vi "DSF.Transceiver.GE Reflective Memory.Initialize Transfer Parameters.vi"(8 "error in (no error)":errorcluster, 10 "Transfer Configurations":refnum<class "DSF.Shared.Configuration.Transfer.lvclass">[](array[class]), 11 "DSF GE Reflective Memory Transceiver in":refnum<class "DSF.Transceiver.GE Reflective Memory.lvclass">) -> (0 "error out":errorcluster, 2 "Transfers Parameters":T1[](array[typedef]) {"size" format="%d bytes"; "offset" format="%08x"}, 3 "DSF GE Reflective Memory Transceiver out":refnum<class "DSF.Transceiver.GE Reflective Memory.lvclass">)   [LabVIEW 2017, in "DSF.Transceiver.GE Reflective Memory.lvlib" / "DSF.Transceiver.GE Reflective Memory.lvclass"]
uses:
  DSF.Transceiver.GE Reflective Memory.lvclass
  DSF Core/Built/Engine/DSF.Engine.lvlibp/Shared/Classes/Transfer/DSF.Shared.Configuration.Transfer.lvclass
  DSF.Transceiver.GE Reflective Memory.Transfer Parameters.ctl
  DSF Core/Built/Engine/DSF.Engine.lvlibp/Shared/Classes/Configuration/DSF.Shared.Configuration.lvclass
  C:/Git/DSF/DSF Core/Built/Engine/DSF.Engine.lvlibp/Shared/Classes/Configuration/DSF.Shared.Configuration.lvclass
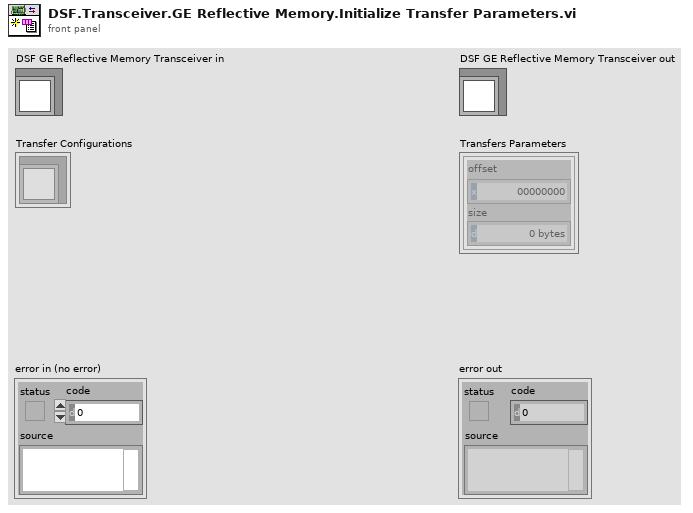
[diagram p1: front panel]
types:
  T1 = typedef "DSF.Transceiver.GE Reflective Memory.lvlib/DSF.Transceiver.GE Reflective Memory.lvclass/DSF.Transceiver.GE Reflective Memory.Transfer Parameters.ctl" = cluster{"offset":u32, "size":u32}
  T2 = typedef "DSF.Engine.lvlibp/DSF Configuration API.lvlib/DSF Settings Info.ctl" = cluster{"key":string, "value":string}[]
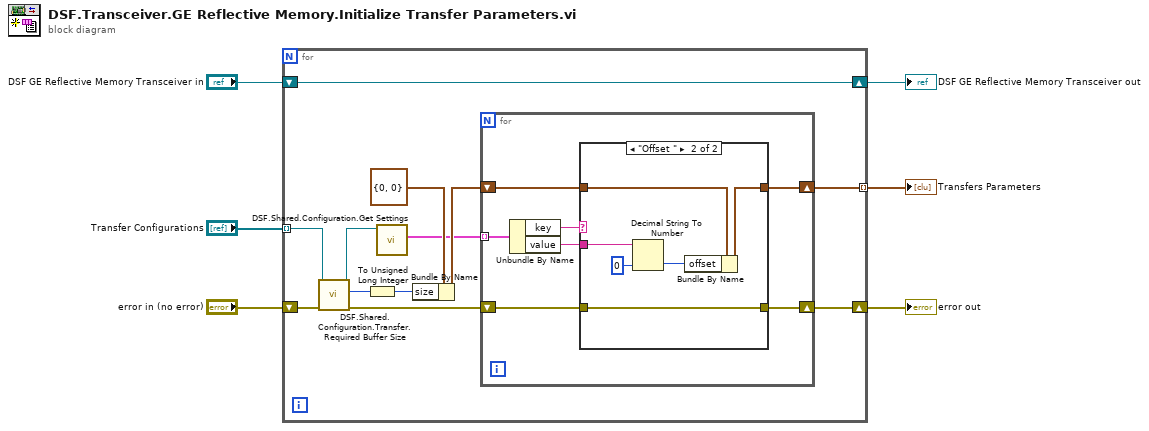
[diagram p0: block diagram]
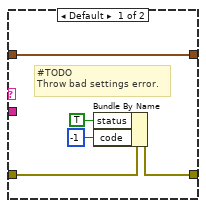
[diagram p2: hidden frame]
diagram:
  n1 = for {
    shift-right: [w10] -> w3
    shift-left: "error in (no error)" -> [w18]
    tunnel: "Transfer Configurations" -> [w9] mode=indexing
    shift-right: [w12] -> w5
    shift-left: "DSF GE Reflective Memory Transceiver in" -> [w12]
    tunnel: [w11] -> w1 mode=indexing
    n2 = call "DSF.Shared.Configuration.Transfer.Required Buffer Size.vi"("error in (no error)"=w18, "Transfer Configuration in"=w9) -> ("error out"=w15:errorcluster, "required buffer size"=w7:u64, "Transfer Configuration out"=w8:refnum<class "DSF.Shared.Configuration.Transfer.lvclass">)  [unwired: 7 in]
    n3 = To Unsigned Long Integer(number=w7) -> (unsigned 32bit integer=w16:u32)
    n4 = call "DSF.Shared.Configuration.Get Settings.vi"("Configuration in"=w8) -> ("settings"=w13:T2)  [unwired: 9 in, 1 out]
    n5 = Bundle By Name(cluster=T1 {"offset"=0, "size"=0} ("Transfer Parameters"), "size"=w16) -> (w17:T1)
    n6 = for {
      shift-right: [w19] -> w10
      shift-left: w15 -> [w25]
      tunnel: w13 -> [w24] mode=indexing
      shift-right: [w20] -> w11
      shift-left: w17 -> [w22]
      n7 = Unbundle By Name(w24) -> ("key"=w23:string, "value"=w21:string)
      n8 = case shown="\"Offset \"" w23 {
        tunnel: w25 -> [w29 w31]
        tunnel: w22 -> [w30 w36]
        tunnel: w21 -> [_ w34]
        tunnel: [w30 w35] -> w20
        tunnel: [w28 w31] -> w19
        frame Default {
          # "#TODO\nThrow bad settings error."
          n9 = Bundle By Name(cluster=w29, "status"=TRUE, "code"=-1) -> (w28:errorcluster)
        }
        frame "Offset " {
          n10 = Decimal String To Number(string=w34, default (0L)=u32 0 ("default (0 I32)")) -> (number=w33:u32)  [unwired: 1 in, 1 out]
          n11 = Bundle By Name(cluster=w36, "offset"=w33) -> (w35:T1)
        }
      }
    }
  }
  "error out" <- w3
  "DSF GE Reflective Memory Transceiver out" <- w5
  "Transfers Parameters" <- w1
